vi "Entrad y salidas dig y analog.vi"() -> ()   [LabVIEW 2017]
uses:
  <vilib>/Instr/_visa.llb/VISA Configure Serial Port (Instr).vi
panel:
  out "BOTON 3":bool
  out "BOTON 2":bool
  out "BOTON 1":bool
  in  "LED 3":bool
  in  "LED 2":bool
  in  "LED 1":bool
  in  "VERDE":i64(knob) scale=0.0..255.0
  in  "ROJO":i64(knob) scale=0.0..255.0
  in  "AZUL":i64(knob) scale=0.0..255.0
  out "POT 3":dbl(knob) scale=0.0..1023.0
  out "POT 2":dbl(knob) scale=0.0..1023.0
  out "POT1":dbl(knob) scale=0.0..1023.0
  in  "VISA resource name":refnum<visa-resource-name>
  # "I/O ANALOGICAS"
  # "I/O DIGITALES"
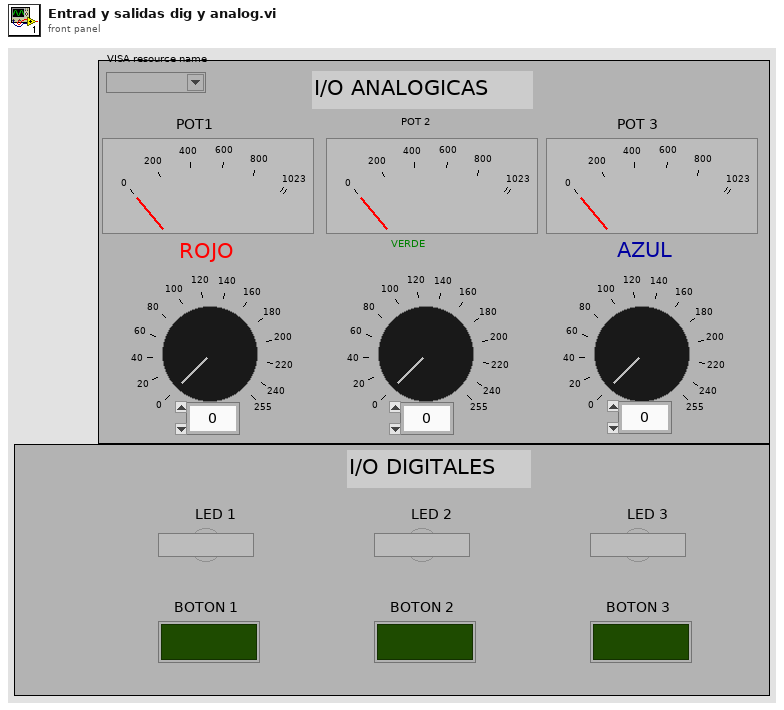
[diagram p1: front panel]
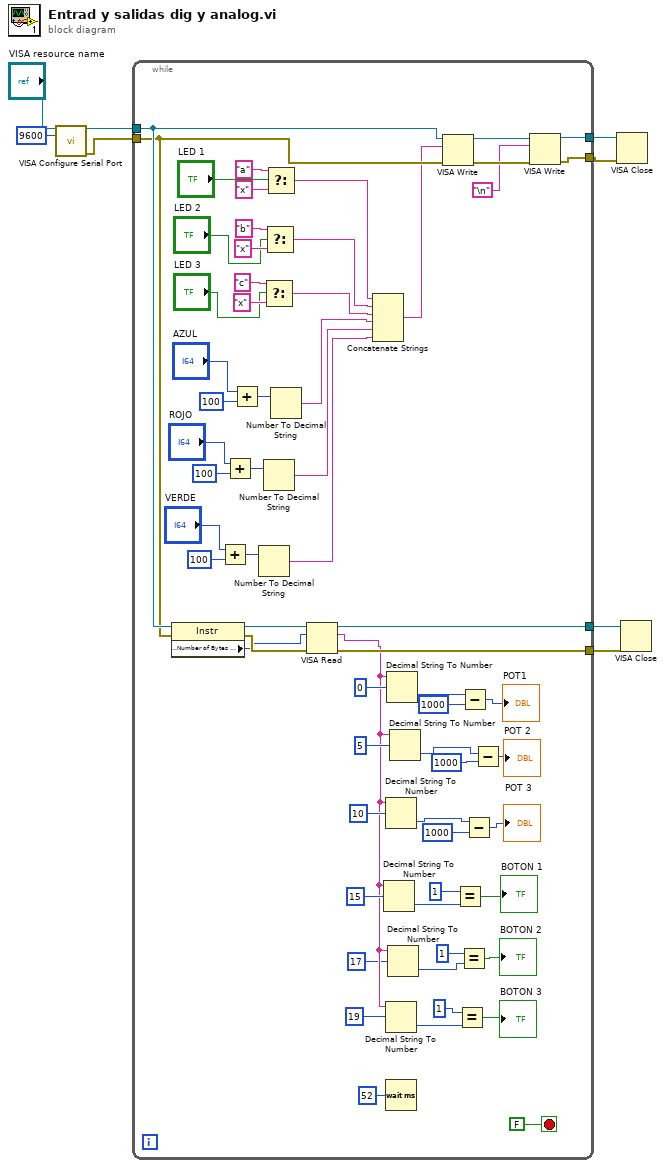
[diagram p0: block diagram]
diagram:
  n1 = call-poly "VISA Configure Serial Port"("VISA resource name"="VISA resource name", "baud rate (9600)"=u32 9600) -> ("VISA resource name out"=w8:refnum<visa-resource-name>, "error out"=w7:errorcluster)  [unwired: 12 in]
  n2 = while {
    tunnel: w8 -> [w21]
    tunnel: w7 -> [w20]
    tunnel: [w28] -> w4
    tunnel: [w27] -> w3
    tunnel: [w26] -> w2
    tunnel: [w25] -> w1
    stop <- FALSE stop-if-true
    n3 = property class="Instr"(reference=w21, error in=w20) -> (reference out=w72:refnum<visa-resource-name>, error out=w71:errorcluster, "Serial Settings:Number of Bytes at Serial Port"=w70:u32)
    n4 = Add(x="VERDE", y=i64 100) -> (x+y=w58:i64)
    n5 = Add(x="ROJO", y=i64 100) -> (x+y=w60:i64)
    n6 = Add(x="AZUL", y=i64 100) -> (x+y=w64:i64)
    n7 = Number To Decimal String(number=w58) -> (decimal integer string=w29:string)  [unwired: 1 in]
    n8 = Select(t="c", s="LED 3", f="x") -> (s? t:f=w32:string)
    n9 = Number To Decimal String(number=w60) -> (decimal integer string=w30:string)  [unwired: 1 in]
    n10 = Select(t="b", s="LED 2", f="x") -> (s? t:f=w33:string)
    n11 = Select(t="a", s="LED 1", f="x") -> (s? t:f=w42:string)
    n12 = Number To Decimal String(number=w64) -> (decimal integer string=w31:string)  [unwired: 1 in]
    n13 = VISA Read(VISA resource name=w72, byte count=w70, error in (no error)=w71) -> (VISA resource name out=w26:refnum<visa-resource-name>, read buffer=w15:string, error out=w25:errorcluster)  [unwired: 1 out]
    n14 = Concatenate Strings(w42, w33, w32, w31, w30, w29) -> (w19:string)
    n15 = Decimal String To Number(string=w15, offset=15 ("offset (0)")) -> (number=w16:i32)  [unwired: 1 in, 1 out]
    n16 = Decimal String To Number(string=w15, offset=10) -> (number=w47:i32)  [unwired: 1 in, 1 out]
    n17 = Decimal String To Number(string=w15, offset=19 ("offset (0)")) -> (number=w9:i32)  [unwired: 1 in, 1 out]
    n18 = Wait (ms)(milliseconds to wait=u32 52) -> ()  [unwired: 1 out]
    n19 = Decimal String To Number(string=w15, offset=0) -> (number=w54:i32)  [unwired: 1 in, 1 out]
    n20 = Decimal String To Number(string=w15, offset=17 ("offset (0)")) -> (number=w11:i32)  [unwired: 1 in, 1 out]
    n21 = Decimal String To Number(string=w15, offset=5) -> (number=w50:i32)  [unwired: 1 in, 1 out]
    n22 = VISA Write(VISA resource name=w21, write buffer=w19, error in (no error)=w20) -> (VISA resource name out=w46:refnum<visa-resource-name>, error out=w45:errorcluster)  [unwired: 1 out]
    n23 = Equal?(x=1 ("y"), y=w16) -> (x = y?=→"BOTON 1":bool)
    n24 = Equal?(x=1 ("y"), y=w9) -> (x = y?=→"BOTON 3":bool)
    n25 = Equal?(x=1 ("y"), y=w11) -> (x = y?=→"BOTON 2":bool)
    n26 = Subtract(x=w54, y=1000) -> (x-y=→"POT1":i32)
    n27 = Subtract(x=w47, y=1000) -> (x-y=→"POT 3":i32)
    n28 = Subtract(x=w50, y=1000) -> (x-y=→"POT 2":i32)
    n29 = VISA Write(VISA resource name=w46, write buffer="\n", error in (no error)=w45) -> (VISA resource name out=w28:refnum<visa-resource-name>, error out=w27:errorcluster)  [unwired: 1 out]
  }
  n30 = VISA Close(VISA resource name=w4, error in (no error)=w3) -> ()  [unwired: 1 out]
  n31 = VISA Close(VISA resource name=w2, error in (no error)=w1) -> ()  [unwired: 1 out]
